vi "Write Icon Data to Library.vi"(8 "error in (no error)":errorcluster, 10 "Data":string, 11 "Library Ref in":refnum<vi>) -> (0 "error out":errorcluster, 3 "Library Ref out":refnum<vi>)   [LabVIEW 2021, in "lv_icon.lvlib"]
doc: "Set the LabVIEW Icon Data of a Library."
uses:
  lv_icon.lvlib
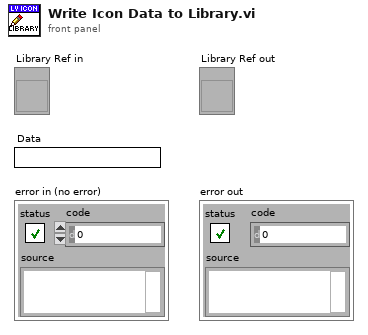
[diagram p1: front panel]
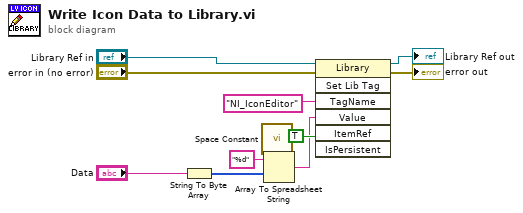
[diagram p0: block diagram]
diagram:
  n1 = String To Byte Array(string="Data") -> (unsigned byte array=w8:u8[])
  n2 = call <vilib>:"Space Constant.vi"() -> ("String"=w5:string)
  n3 = Array To Spreadsheet String(delimiter (Tab)=w5, array=w8, 3:"%d" ("format string")) -> (spreadsheet string=w6:string)
  n4 = invoke class="Library" method="Set Lib Tag"(reference="Library Ref in", error in="error in (no error)", "TagName"="NI_IconEditor" ("Tag Name"), "Value"=w6, "ItemRef"=TRUE ("Is Persistent")) -> (reference out=→"Library Ref out":refnum<vi>, error out=→"error out":errorcluster)  [unwired: 2 in, 5 out]
